vi "SelectOPCTags.GetChannelInfo.vi"(8 "error in (no error)":errorcluster, 10 "Item URL":string, 11 "OPC UA client refnum in":refnum<k21>) -> (0 "error out":errorcluster, 1 "Setings":T1={"Settings"={"name"="", "node type"=enum."Other", "DataType"=1, "access"=enum."Null", "description"=""}, "Array Size"=0} {"Settings"."DataType" items=["Boolean"=1, "SByte"=2, "Byte"=3, "Int16"=4, "UInt16"=5, "Int32"=6, "UInt32"=7, "Int64"=8, "UInt64"=9, "Float"=10, "Double"=11, "String"=12, "DateTime"=13, "ByteString"=15, "Array of Boolean"=101, "Array of SByte"=102, "Array of Byte"=103, "Array of Int16"=104, "Array of UInt16"=105, "Array of Int32"=106, "Array of UInt32"=107, "Array of Int64"=108, "Array of UInt64"=109, "Array of Float"=110, "Array of Double"=111, "Array of String"=112, "Array of DateTime"=113, "Array of ByteString"=115]}, 2 "Item URL out":string, 3 "OPC UA client refnum out":refnum<k21>, 4 "Use":bool)   [LabVIEW 2019, in "OPC UA Client System Explorer.lvlib"]
uses:
  OPC UA Client System Explorer.lvlib
  Types/Tag.TreeSettings.ctl
  <vilib>/OPCUA/NI OPC UA Client.lvlib
  <vilib>/OPCUA/client/internal/Read Double Array.vi
  <vilib>/OPCUA/client/internal/Read Float Array.vi
  <vilib>/OPCUA/client/internal/Read UInt32 Array.vi
  <vilib>/OPCUA/client/internal/Read Int32 Array.vi
  <vilib>/OPCUA/client/internal/Read UInt16 Array.vi
  <vilib>/OPCUA/client/internal/Read Int16 Array.vi
  <vilib>/OPCUA/client/internal/Read Byte Array.vi
  <vilib>/OPCUA/client/internal/Read SByte Array.vi
  <vilib>/OPCUA/client/internal/Read Bool Array.vi
  <vilib>/OPCUA/client/internal/Read UInt64 Array.vi
  <vilib>/OPCUA/client/internal/Read Int64 Array.vi
  <vilib>/OPCUA/client/internal/Read DateTime Array.vi
  <vilib>/OPCUA/client/internal/Read ByteString.vi
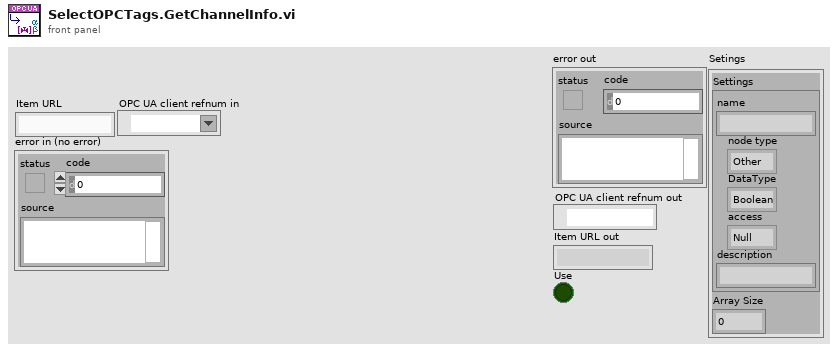
[diagram p1: front panel]
types:
  T1 = typedef "OPC UA Client System Explorer.lvlib/Tag.TreeSettings.ctl" = cluster{"Settings":cluster{"name":string, "node type":enum32{"Other", "Folder", "Item/Property"}, "DataType":u32, "access":enum16{"Null", "Read", "Write", "Read&Write"}, "description":string}, "Array Size":i32}
  T2 = typedef "Data Type Indicator.ctl" = u16
  T3 = cluster{"name":string, "node class":u16, "data type":T2, "access":enum16{"Null", "Read", "Write", "Read&Write"}, "description":string}
  T4 = typedef "OPC UA Client Refnum.ctl" = refnum<k21>
  T5 = typedef "OPC UA StatusCode.ctl" = u32
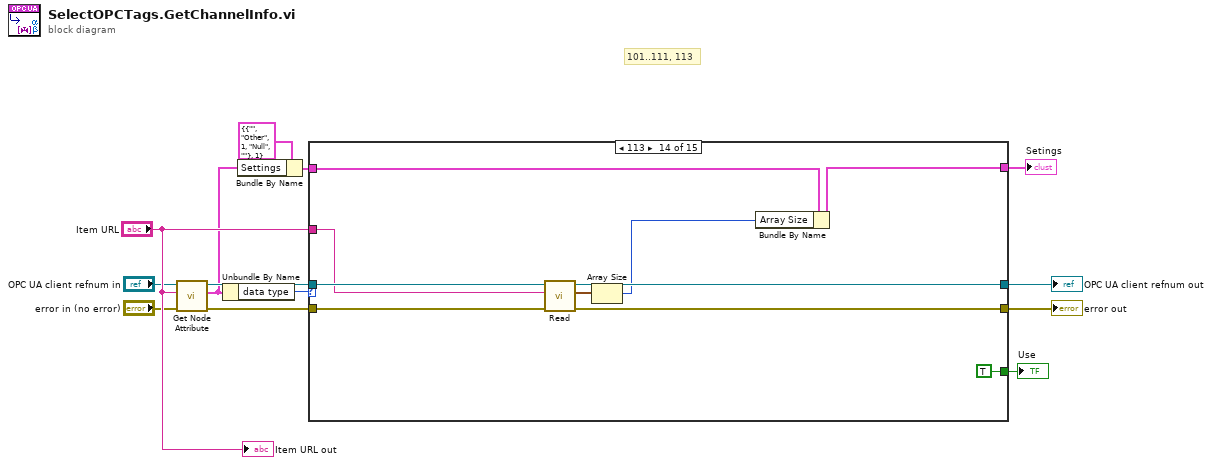
[diagram p0: block diagram]
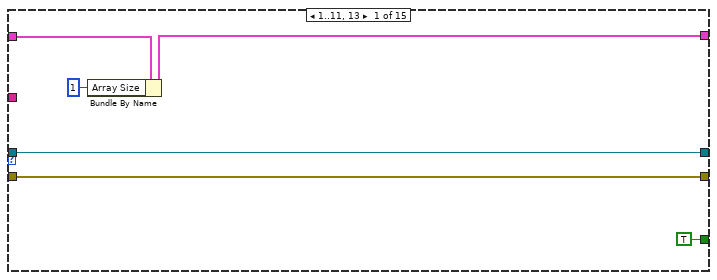
[diagram p2: hidden frame]
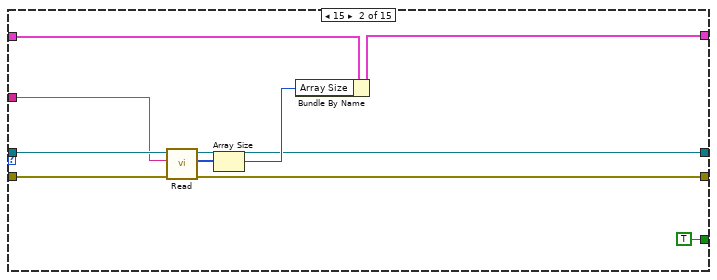
[diagram p3: hidden frame]
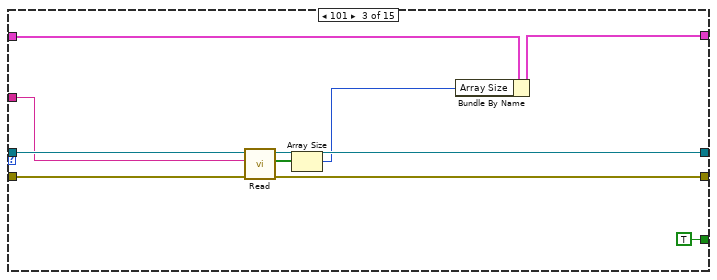
[diagram p4: hidden frame]
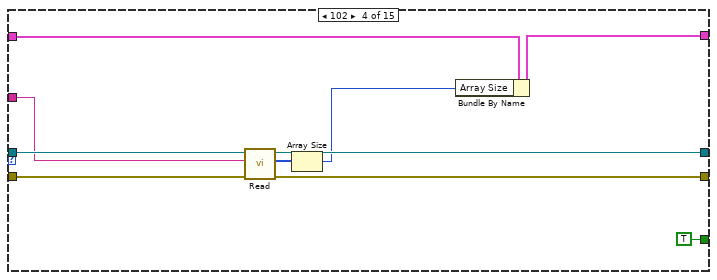
[diagram p5: hidden frame]
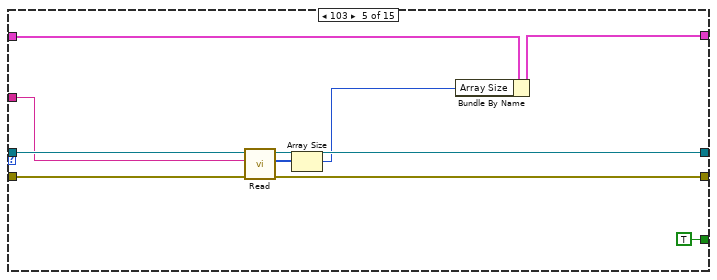
[diagram p6: hidden frame]
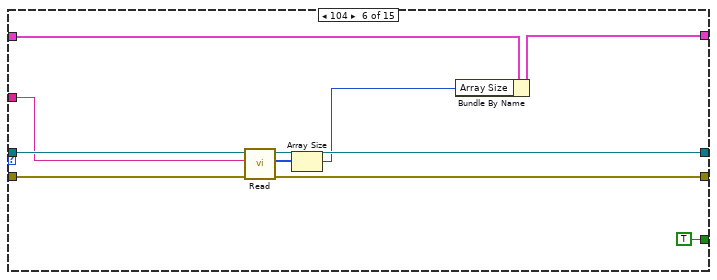
[diagram p7: hidden frame]
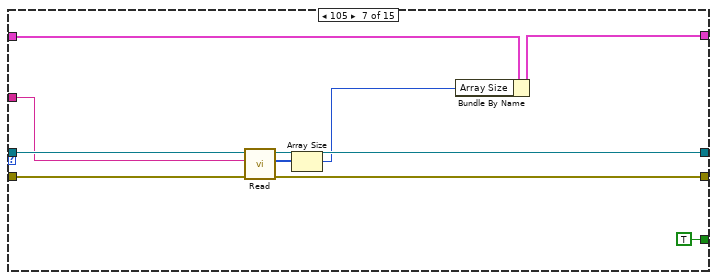
[diagram p8: hidden frame]
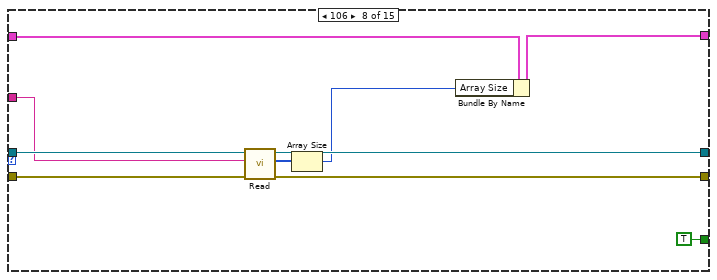
[diagram p9: hidden frame]
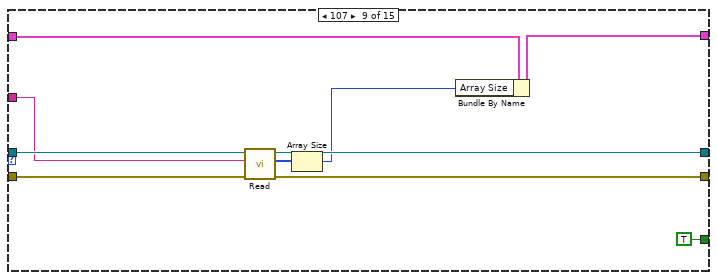
[diagram p10: hidden frame]
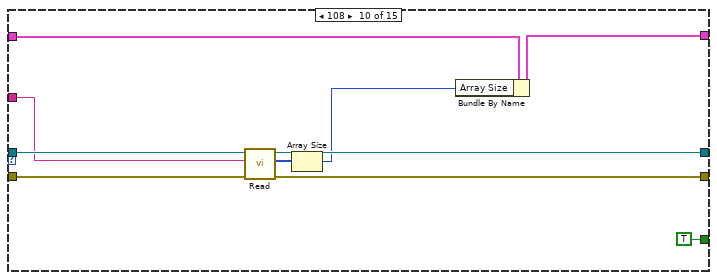
[diagram p11: hidden frame]
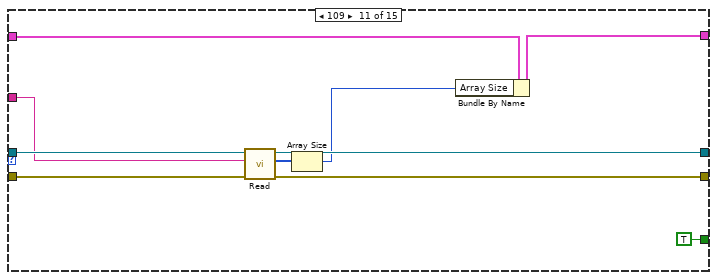
[diagram p12: hidden frame]
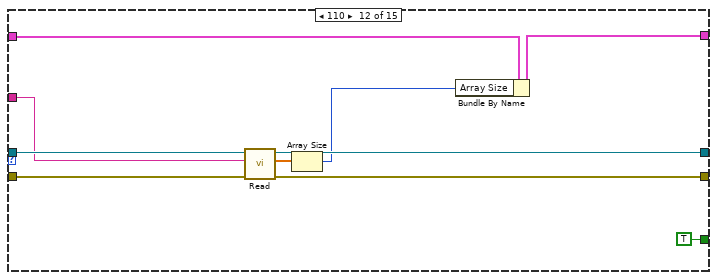
[diagram p13: hidden frame]
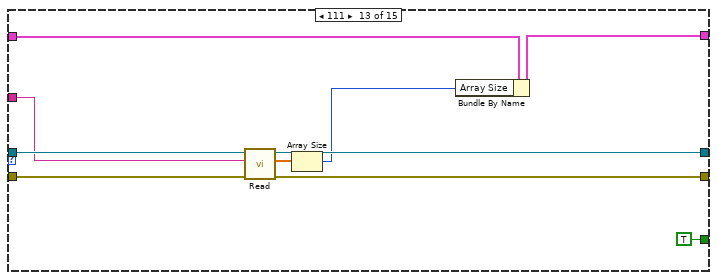
[diagram p14: hidden frame]
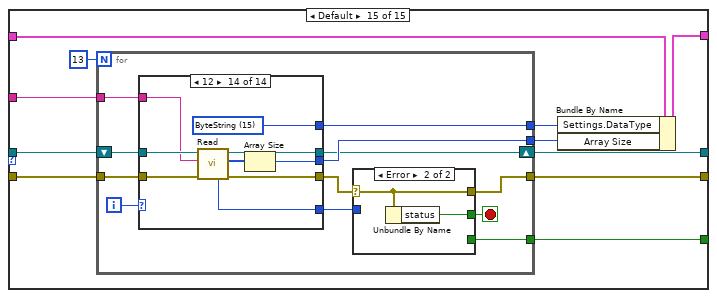
[diagram p15: hidden frame]
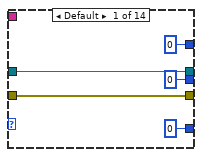
[diagram p16: hidden frame]
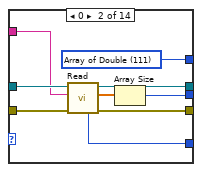
[diagram p17: hidden frame]
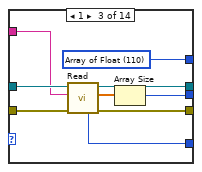
[diagram p18: hidden frame]
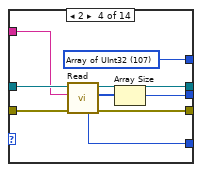
[diagram p19: hidden frame]
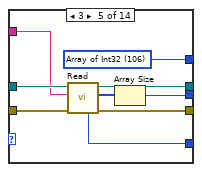
[diagram p20: hidden frame]
diagram:
  # "101..111, 113"
  n1 = call <vilib>:"Get Node Attribute.vi"("error in (no error)"="error in (no error)", "node ID"="Item URL", "OPC UA client refnum in"="OPC UA client refnum in") -> ("error out"=w6:errorcluster, "node attribute"=w4:T3, "OPC UA client refnum out"=w5:T4)  [unwired: 5 in, 1 out]
  n2 = Unbundle By Name(w4) -> ("data type"=w10:T2)
  n3 = Bundle By Name(cluster=T1 {"Settings"={"name"="", "node type"=enum."Other", "DataType"=1, "access"=enum."Null", "description"=""}, "Array Size"=1}, "Settings"=w4) -> (w9:T1)
  n4 = case shown="113" w10 {
    tunnel: [w16 w20 w34 w44 w54 w64 w74 w84 w94 w104 w114 w124 w134 w144 w152] -> w13
    tunnel: [w17 w21 w32 w42 w52 w62 w72 w82 w92 w102 w112 w122 w132 w142 w151] -> w12
    tunnel: w6 -> [w16 w25 w35 w45 w55 w65 w75 w85 w95 w105 w115 w125 w135 w145 w157]
    tunnel: w5 -> [w17 w24 w33 w43 w53 w63 w73 w83 w93 w103 w113 w123 w133 w143 w155]
    tunnel: "Item URL" -> [_ w23 w30 w40 w50 w60 w70 w80 w90 w100 w110 w120 w130 w140 w156]
    tunnel: w9 -> [w19 w29 w39 w49 w59 w69 w79 w89 w99 w109 w119 w129 w139 w149 w160]
    tunnel: [w18 w28 w38 w48 w58 w68 w78 w88 w98 w108 w118 w128 w138 w148 w159] -> w3
    tunnel: [TRUE ("status") TRUE ("status") TRUE ("status") TRUE ("status") TRUE ("status") TRUE ("status") TRUE ("status") TRUE ("status") TRUE ("status") TRUE ("status") TRUE ("status") TRUE ("status") TRUE ("status") TRUE ("status") w150] -> w2
    frame 1..11, 13 {
      n5 = Bundle By Name(cluster=w19, "Array Size"=1) -> (w18:T1)
    }
    frame 15 {
      n6 = call-poly <vilib>:"Read.vi"("error in (no error)"=w25, "node ID"=w23, "OPC UA client refnum in"=w24) -> ("error out"=w20:errorcluster, "value"=w26:u8[], "OPC UA client refnum out"=w21:T4)  [unwired: 4 in, 2 out]
      n7 = Array Size(array=w26) -> (size(s)=w22:i32)
      n8 = Bundle By Name(cluster=w29, "Array Size"=w22) -> (w28:T1)
    }
    frame 101 {
      n9 = call-poly <vilib>:"Read.vi"("error in (no error)"=w35, "node ID"=w30, "OPC UA client refnum in"=w33) -> ("error out"=w34:errorcluster, "values"=w36:bool[], "OPC UA client refnum out"=w32:T4)  [unwired: 4 in, 2 out]
      n10 = Array Size(array=w36) -> (size(s)=w31:i32)
      n11 = Bundle By Name(cluster=w39, "Array Size"=w31) -> (w38:T1)
    }
    frame 102 {
      n12 = call-poly <vilib>:"Read.vi"("error in (no error)"=w45, "node ID"=w40, "OPC UA client refnum in"=w43) -> ("error out"=w44:errorcluster, "values"=w46:i8[], "OPC UA client refnum out"=w42:T4)  [unwired: 4 in, 2 out]
      n13 = Array Size(array=w46) -> (size(s)=w41:i32)
      n14 = Bundle By Name(cluster=w49, "Array Size"=w41) -> (w48:T1)
    }
    frame 103 {
      n15 = call-poly <vilib>:"Read.vi"("error in (no error)"=w55, "node ID"=w50, "OPC UA client refnum in"=w53) -> ("error out"=w54:errorcluster, "values"=w56:u8[], "OPC UA client refnum out"=w52:T4)  [unwired: 4 in, 2 out]
      n16 = Array Size(array=w56) -> (size(s)=w51:i32)
      n17 = Bundle By Name(cluster=w59, "Array Size"=w51) -> (w58:T1)
    }
    frame 104 {
      n18 = call-poly <vilib>:"Read.vi"("error in (no error)"=w65, "node ID"=w60, "OPC UA client refnum in"=w63) -> ("error out"=w64:errorcluster, "values"=w66:i16[], "OPC UA client refnum out"=w62:T4)  [unwired: 4 in, 2 out]
      n19 = Array Size(array=w66) -> (size(s)=w61:i32)
      n20 = Bundle By Name(cluster=w69, "Array Size"=w61) -> (w68:T1)
    }
    frame 105 {
      n21 = call-poly <vilib>:"Read.vi"("error in (no error)"=w75, "node ID"=w70, "OPC UA client refnum in"=w73) -> ("error out"=w74:errorcluster, "values"=w76:u16[], "OPC UA client refnum out"=w72:T4)  [unwired: 4 in, 2 out]
      n22 = Array Size(array=w76) -> (size(s)=w71:i32)
      n23 = Bundle By Name(cluster=w79, "Array Size"=w71) -> (w78:T1)
    }
    frame 106 {
      n24 = call-poly <vilib>:"Read.vi"("error in (no error)"=w85, "node ID"=w80, "OPC UA client refnum in"=w83) -> ("error out"=w84:errorcluster, "values"=w86:i32[], "OPC UA client refnum out"=w82:T4)  [unwired: 4 in, 2 out]
      n25 = Array Size(array=w86) -> (size(s)=w81:i32)
      n26 = Bundle By Name(cluster=w89, "Array Size"=w81) -> (w88:T1)
    }
    frame 107 {
      n27 = call-poly <vilib>:"Read.vi"("error in (no error)"=w95, "node ID"=w90, "OPC UA client refnum in"=w93) -> ("error out"=w94:errorcluster, "values"=w96:u32[], "OPC UA client refnum out"=w92:T4)  [unwired: 4 in, 2 out]
      n28 = Array Size(array=w96) -> (size(s)=w91:i32)
      n29 = Bundle By Name(cluster=w99, "Array Size"=w91) -> (w98:T1)
    }
    frame 108 {
      n30 = call-poly <vilib>:"Read.vi"("error in (no error)"=w105, "node ID"=w100, "OPC UA client refnum in"=w103) -> ("error out"=w104:errorcluster, "values"=w106:i64[], "OPC UA client refnum out"=w102:T4)  [unwired: 4 in, 2 out]
      n31 = Array Size(array=w106) -> (size(s)=w101:i32)
      n32 = Bundle By Name(cluster=w109, "Array Size"=w101) -> (w108:T1)
    }
    frame 109 {
      n33 = call-poly <vilib>:"Read.vi"("error in (no error)"=w115, "node ID"=w110, "OPC UA client refnum in"=w113) -> ("error out"=w114:errorcluster, "values"=w116:u64[], "OPC UA client refnum out"=w112:T4)  [unwired: 4 in, 2 out]
      n34 = Array Size(array=w116) -> (size(s)=w111:i32)
      n35 = Bundle By Name(cluster=w119, "Array Size"=w111) -> (w118:T1)
    }
    frame 110 {
      n36 = call-poly <vilib>:"Read.vi"("error in (no error)"=w125, "node ID"=w120, "OPC UA client refnum in"=w123) -> ("error out"=w124:errorcluster, "values"=w126:sgl[], "OPC UA client refnum out"=w122:T4)  [unwired: 4 in, 2 out]
      n37 = Array Size(array=w126) -> (size(s)=w121:i32)
      n38 = Bundle By Name(cluster=w129, "Array Size"=w121) -> (w128:T1)
    }
    frame 111 {
      n39 = call-poly <vilib>:"Read.vi"("error in (no error)"=w135, "node ID"=w130, "OPC UA client refnum in"=w133) -> ("error out"=w134:errorcluster, "values"=w136:dbl[], "OPC UA client refnum out"=w132:T4)  [unwired: 4 in, 2 out]
      n40 = Array Size(array=w136) -> (size(s)=w131:i32)
      n41 = Bundle By Name(cluster=w139, "Array Size"=w131) -> (w138:T1)
    }
    frame 113 {
      n42 = call-poly <vilib>:"Read.vi"("error in (no error)"=w145, "node ID"=w140, "OPC UA client refnum in"=w143) -> ("error out"=w144:errorcluster, "values"=w146:timestamp[], "OPC UA client refnum out"=w142:T4)  [unwired: 4 in, 2 out]
      n43 = Array Size(array=w146) -> (size(s)=w141:i32)
      n44 = Bundle By Name(cluster=w149, "Array Size"=w141) -> (w148:T1)
    }
    frame Default {
      n45 = for {
        N: 13 -> [_]
        tunnel: w157 -> [w172]
        tunnel: w156 -> [w170]
        tunnel: [w167] -> w152
        tunnel: [w165] -> w153
        tunnel: [w164] -> w154
        shift-right: [w163] -> w151
        shift-left: w155 -> [w171]
        tunnel: [w161] -> w150
        i -> [w166]
        stop <- w162 stop-if-true
        n46 = case shown="12" w166 {
          tunnel: w172 -> [w175 w186 w195 w204 w213 w222 w231 w240 w249 w258 w267 w276 w285 w294]
          tunnel: w171 -> [w173 w185 w194 w203 w212 w221 w230 w239 w248 w257 w266 w275 w284 w293]
          tunnel: w170 -> [_ w184 w193 w202 w211 w220 w229 w238 w247 w256 w265 w274 w283 w292]
          tunnel: [w175 w183 w192 w201 w210 w219 w228 w237 w246 w255 w264 w273 w282 w291] -> w169
          tunnel: [u32 0 ("status") w182 w191 w200 w209 w218 w227 w236 w245 w254 w263 w272 w281 w290] -> w168
          tunnel: [u32 0 ("DataType") w180 w189 w198 w207 w216 w225 w234 w243 w252 w261 w270 w279 w288] -> w164
          tunnel: [0 w179 w188 w197 w206 w215 w224 w233 w242 w251 w260 w269 w278 w287] -> w165
          tunnel: [w173 w178 w187 w196 w205 w214 w223 w232 w241 w250 w259 w268 w277 w286] -> w163
          frame Default {
          }
          frame 0 {
            w180 = u32 111 items=["Boolean"=1, "SByte"=2, "Byte"=3, "Int16"=4, "UInt16"=5, "Int32"=6, "UInt32"=7, "Int64"=8, "UInt64"=9, "Float"=10, "Double"=11, "String"=12, "DateTime"=13, "ByteString"=15, "Array of Boolean"=101, "Array of SByte"=102, "Array of Byte"=103, "Array of Int16"=104, "Array of UInt16"=105, "Array of Int32"=106, "Array of UInt32"=107, "Array of Int64"=108, "Array of UInt64"=109, "Array of Float"=110, "Array of Double"=111, "Array of String"=112, "Array of DateTime"=113, "Array of ByteString"=115] ("DataType")
            n47 = call-poly <vilib>:"Read.vi"("error in (no error)"=w186, "node ID"=w184, "OPC UA client refnum in"=w185) -> ("error out"=w183:errorcluster, "values"=w181:dbl[], "OPC UA client refnum out"=w178:T4, "status"=w182:T5)  [unwired: 4 in, 1 out]
            n48 = Array Size(array=w181) -> (size(s)=w179:i32)
          }
          frame 1 {
            w189 = u32 110 items=["Boolean"=1, "SByte"=2, "Byte"=3, "Int16"=4, "UInt16"=5, "Int32"=6, "UInt32"=7, "Int64"=8, "UInt64"=9, "Float"=10, "Double"=11, "String"=12, "DateTime"=13, "ByteString"=15, "Array of Boolean"=101, "Array of SByte"=102, "Array of Byte"=103, "Array of Int16"=104, "Array of UInt16"=105, "Array of Int32"=106, "Array of UInt32"=107, "Array of Int64"=108, "Array of UInt64"=109, "Array of Float"=110, "Array of Double"=111, "Array of String"=112, "Array of DateTime"=113, "Array of ByteString"=115] ("DataType")
            n49 = call-poly <vilib>:"Read.vi"("error in (no error)"=w195, "node ID"=w193, "OPC UA client refnum in"=w194) -> ("error out"=w192:errorcluster, "values"=w190:sgl[], "OPC UA client refnum out"=w187:T4, "status"=w191:T5)  [unwired: 4 in, 1 out]
            n50 = Array Size(array=w190) -> (size(s)=w188:i32)
          }
          frame 2 {
            w198 = u32 107 items=["Boolean"=1, "SByte"=2, "Byte"=3, "Int16"=4, "UInt16"=5, "Int32"=6, "UInt32"=7, "Int64"=8, "UInt64"=9, "Float"=10, "Double"=11, "String"=12, "DateTime"=13, "ByteString"=15, "Array of Boolean"=101, "Array of SByte"=102, "Array of Byte"=103, "Array of Int16"=104, "Array of UInt16"=105, "Array of Int32"=106, "Array of UInt32"=107, "Array of Int64"=108, "Array of UInt64"=109, "Array of Float"=110, "Array of Double"=111, "Array of String"=112, "Array of DateTime"=113, "Array of ByteString"=115] ("DataType")
            n51 = call-poly <vilib>:"Read.vi"("error in (no error)"=w204, "node ID"=w202, "OPC UA client refnum in"=w203) -> ("error out"=w201:errorcluster, "values"=w199:u32[], "OPC UA client refnum out"=w196:T4, "status"=w200:T5)  [unwired: 4 in, 1 out]
            n52 = Array Size(array=w199) -> (size(s)=w197:i32)
          }
          frame 3 {
            w207 = u32 106 items=["Boolean"=1, "SByte"=2, "Byte"=3, "Int16"=4, "UInt16"=5, "Int32"=6, "UInt32"=7, "Int64"=8, "UInt64"=9, "Float"=10, "Double"=11, "String"=12, "DateTime"=13, "ByteString"=15, "Array of Boolean"=101, "Array of SByte"=102, "Array of Byte"=103, "Array of Int16"=104, "Array of UInt16"=105, "Array of Int32"=106, "Array of UInt32"=107, "Array of Int64"=108, "Array of UInt64"=109, "Array of Float"=110, "Array of Double"=111, "Array of String"=112, "Array of DateTime"=113, "Array of ByteString"=115] ("DataType")
            n53 = call-poly <vilib>:"Read.vi"("error in (no error)"=w213, "node ID"=w211, "OPC UA client refnum in"=w212) -> ("error out"=w210:errorcluster, "values"=w208:i32[], "OPC UA client refnum out"=w205:T4, "status"=w209:T5)  [unwired: 4 in, 1 out]
            n54 = Array Size(array=w208) -> (size(s)=w206:i32)
          }
          frame 4 {
            w216 = u32 105 items=["Boolean"=1, "SByte"=2, "Byte"=3, "Int16"=4, "UInt16"=5, "Int32"=6, "UInt32"=7, "Int64"=8, "UInt64"=9, "Float"=10, "Double"=11, "String"=12, "DateTime"=13, "ByteString"=15, "Array of Boolean"=101, "Array of SByte"=102, "Array of Byte"=103, "Array of Int16"=104, "Array of UInt16"=105, "Array of Int32"=106, "Array of UInt32"=107, "Array of Int64"=108, "Array of UInt64"=109, "Array of Float"=110, "Array of Double"=111, "Array of String"=112, "Array of DateTime"=113, "Array of ByteString"=115] ("DataType")
            n55 = call-poly <vilib>:"Read.vi"("error in (no error)"=w222, "node ID"=w220, "OPC UA client refnum in"=w221) -> ("error out"=w219:errorcluster, "values"=w217:u16[], "OPC UA client refnum out"=w214:T4, "status"=w218:T5)  [unwired: 4 in, 1 out]
            n56 = Array Size(array=w217) -> (size(s)=w215:i32)
          }
          frame 5 {
            w225 = u32 104 items=["Boolean"=1, "SByte"=2, "Byte"=3, "Int16"=4, "UInt16"=5, "Int32"=6, "UInt32"=7, "Int64"=8, "UInt64"=9, "Float"=10, "Double"=11, "String"=12, "DateTime"=13, "ByteString"=15, "Array of Boolean"=101, "Array of SByte"=102, "Array of Byte"=103, "Array of Int16"=104, "Array of UInt16"=105, "Array of Int32"=106, "Array of UInt32"=107, "Array of Int64"=108, "Array of UInt64"=109, "Array of Float"=110, "Array of Double"=111, "Array of String"=112, "Array of DateTime"=113, "Array of ByteString"=115] ("DataType")
            n57 = call-poly <vilib>:"Read.vi"("error in (no error)"=w231, "node ID"=w229, "OPC UA client refnum in"=w230) -> ("error out"=w228:errorcluster, "values"=w226:i16[], "OPC UA client refnum out"=w223:T4, "status"=w227:T5)  [unwired: 4 in, 1 out]
            n58 = Array Size(array=w226) -> (size(s)=w224:i32)
          }
          frame 6 {
            w234 = u32 103 items=["Boolean"=1, "SByte"=2, "Byte"=3, "Int16"=4, "UInt16"=5, "Int32"=6, "UInt32"=7, "Int64"=8, "UInt64"=9, "Float"=10, "Double"=11, "String"=12, "DateTime"=13, "ByteString"=15, "Array of Boolean"=101, "Array of SByte"=102, "Array of Byte"=103, "Array of Int16"=104, "Array of UInt16"=105, "Array of Int32"=106, "Array of UInt32"=107, "Array of Int64"=108, "Array of UInt64"=109, "Array of Float"=110, "Array of Double"=111, "Array of String"=112, "Array of DateTime"=113, "Array of ByteString"=115] ("DataType")
            n59 = call-poly <vilib>:"Read.vi"("error in (no error)"=w240, "node ID"=w238, "OPC UA client refnum in"=w239) -> ("error out"=w237:errorcluster, "values"=w235:u8[], "OPC UA client refnum out"=w232:T4, "status"=w236:T5)  [unwired: 4 in, 1 out]
            n60 = Array Size(array=w235) -> (size(s)=w233:i32)
          }
          frame 7 {
            w243 = u32 102 items=["Boolean"=1, "SByte"=2, "Byte"=3, "Int16"=4, "UInt16"=5, "Int32"=6, "UInt32"=7, "Int64"=8, "UInt64"=9, "Float"=10, "Double"=11, "String"=12, "DateTime"=13, "ByteString"=15, "Array of Boolean"=101, "Array of SByte"=102, "Array of Byte"=103, "Array of Int16"=104, "Array of UInt16"=105, "Array of Int32"=106, "Array of UInt32"=107, "Array of Int64"=108, "Array of UInt64"=109, "Array of Float"=110, "Array of Double"=111, "Array of String"=112, "Array of DateTime"=113, "Array of ByteString"=115] ("DataType")
            n61 = call-poly <vilib>:"Read.vi"("error in (no error)"=w249, "node ID"=w247, "OPC UA client refnum in"=w248) -> ("error out"=w246:errorcluster, "values"=w244:i8[], "OPC UA client refnum out"=w241:T4, "status"=w245:T5)  [unwired: 4 in, 1 out]
            n62 = Array Size(array=w244) -> (size(s)=w242:i32)
          }
          frame 8 {
            w252 = u32 101 items=["Boolean"=1, "SByte"=2, "Byte"=3, "Int16"=4, "UInt16"=5, "Int32"=6, "UInt32"=7, "Int64"=8, "UInt64"=9, "Float"=10, "Double"=11, "String"=12, "DateTime"=13, "ByteString"=15, "Array of Boolean"=101, "Array of SByte"=102, "Array of Byte"=103, "Array of Int16"=104, "Array of UInt16"=105, "Array of Int32"=106, "Array of UInt32"=107, "Array of Int64"=108, "Array of UInt64"=109, "Array of Float"=110, "Array of Double"=111, "Array of String"=112, "Array of DateTime"=113, "Array of ByteString"=115] ("DataType")
            n63 = call-poly <vilib>:"Read.vi"("error in (no error)"=w258, "node ID"=w256, "OPC UA client refnum in"=w257) -> ("error out"=w255:errorcluster, "values"=w253:bool[], "OPC UA client refnum out"=w250:T4, "status"=w254:T5)  [unwired: 4 in, 1 out]
            n64 = Array Size(array=w253) -> (size(s)=w251:i32)
          }
          frame 9 {
            w261 = u32 109 items=["Boolean"=1, "SByte"=2, "Byte"=3, "Int16"=4, "UInt16"=5, "Int32"=6, "UInt32"=7, "Int64"=8, "UInt64"=9, "Float"=10, "Double"=11, "String"=12, "DateTime"=13, "ByteString"=15, "Array of Boolean"=101, "Array of SByte"=102, "Array of Byte"=103, "Array of Int16"=104, "Array of UInt16"=105, "Array of Int32"=106, "Array of UInt32"=107, "Array of Int64"=108, "Array of UInt64"=109, "Array of Float"=110, "Array of Double"=111, "Array of String"=112, "Array of DateTime"=113, "Array of ByteString"=115] ("DataType")
            n65 = call-poly <vilib>:"Read.vi"("error in (no error)"=w267, "node ID"=w265, "OPC UA client refnum in"=w266) -> ("error out"=w264:errorcluster, "values"=w262:u64[], "OPC UA client refnum out"=w259:T4, "status"=w263:T5)  [unwired: 4 in, 1 out]
            n66 = Array Size(array=w262) -> (size(s)=w260:i32)
          }
          frame 10 {
            w270 = u32 108 items=["Boolean"=1, "SByte"=2, "Byte"=3, "Int16"=4, "UInt16"=5, "Int32"=6, "UInt32"=7, "Int64"=8, "UInt64"=9, "Float"=10, "Double"=11, "String"=12, "DateTime"=13, "ByteString"=15, "Array of Boolean"=101, "Array of SByte"=102, "Array of Byte"=103, "Array of Int16"=104, "Array of UInt16"=105, "Array of Int32"=106, "Array of UInt32"=107, "Array of Int64"=108, "Array of UInt64"=109, "Array of Float"=110, "Array of Double"=111, "Array of String"=112, "Array of DateTime"=113, "Array of ByteString"=115] ("DataType")
            n67 = call-poly <vilib>:"Read.vi"("error in (no error)"=w276, "node ID"=w274, "OPC UA client refnum in"=w275) -> ("error out"=w273:errorcluster, "values"=w271:i64[], "OPC UA client refnum out"=w268:T4, "status"=w272:T5)  [unwired: 4 in, 1 out]
            n68 = Array Size(array=w271) -> (size(s)=w269:i32)
          }
          frame 11 {
            w279 = u32 113 items=["Boolean"=1, "SByte"=2, "Byte"=3, "Int16"=4, "UInt16"=5, "Int32"=6, "UInt32"=7, "Int64"=8, "UInt64"=9, "Float"=10, "Double"=11, "String"=12, "DateTime"=13, "ByteString"=15, "Array of Boolean"=101, "Array of SByte"=102, "Array of Byte"=103, "Array of Int16"=104, "Array of UInt16"=105, "Array of Int32"=106, "Array of UInt32"=107, "Array of Int64"=108, "Array of UInt64"=109, "Array of Float"=110, "Array of Double"=111, "Array of String"=112, "Array of DateTime"=113, "Array of ByteString"=115] ("DataType")
            n69 = call-poly <vilib>:"Read.vi"("error in (no error)"=w285, "node ID"=w283, "OPC UA client refnum in"=w284) -> ("error out"=w282:errorcluster, "values"=w280:timestamp[], "OPC UA client refnum out"=w277:T4, "status"=w281:T5)  [unwired: 4 in, 1 out]
            n70 = Array Size(array=w280) -> (size(s)=w278:i32)
          }
          frame 12 {
            w288 = u32 15 items=["Boolean"=1, "SByte"=2, "Byte"=3, "Int16"=4, "UInt16"=5, "Int32"=6, "UInt32"=7, "Int64"=8, "UInt64"=9, "Float"=10, "Double"=11, "String"=12, "DateTime"=13, "ByteString"=15, "Array of Boolean"=101, "Array of SByte"=102, "Array of Byte"=103, "Array of Int16"=104, "Array of UInt16"=105, "Array of Int32"=106, "Array of UInt32"=107, "Array of Int64"=108, "Array of UInt64"=109, "Array of Float"=110, "Array of Double"=111, "Array of String"=112, "Array of DateTime"=113, "Array of ByteString"=115] ("DataType")
            n71 = call-poly <vilib>:"Read.vi"("error in (no error)"=w294, "node ID"=w292, "OPC UA client refnum in"=w293) -> ("error out"=w291:errorcluster, "value"=w289:u8[], "OPC UA client refnum out"=w286:T4, "status"=w290:T5)  [unwired: 4 in, 1 out]
            n72 = Array Size(array=w289) -> (size(s)=w287:i32)
          }
        }
        n73 = case shown="Error" w169 {
          selector: w169 -> [w296 w299]
          tunnel: w168 -> [w298 _]
          tunnel: [w295 w300] -> w162
          tunnel: [w296 w299] -> w167
          tunnel: [w295 _] -> w161
          frame No Error {
            w297 = u32 0 items=["Good"=0, "Bad_AttributeIdInvalid"=2153906176, "Bad_BrowseDirectionInvalid"=2152529920, "Bad_BrowseNameInvalid"=2153775104, "Bad_ContentFilterInvalid"=2152202240, "Bad_ContinuationPointInvalid"=2152333312, "Bad_DataEncodingInvalid"=2151153664, "Bad_DataEncodingUnsupported"=2151219200, "Bad_EventFilterInvalid"=2152136704, "Bad_FilterNotAllowed"=2152005632, "Bad_FilterOperandInvalid"=2160132096, "Bad_HistoryOperationInvalid"=2154889216, "Bad_HistoryOperationUnsupported"=2154954752, "Bad_IndexRangeInvalid"=2151022592, "Bad_IndexRangeNoData"=2151088128, "Bad_MonitoredItemFilterInvalid"=2151874560, "Bad_MonitoredItemFilterUnsupported"=2151940096, "Bad_MonitoredItemIdInvalid"=2151809024, "Bad_MonitoringModeInvalid"=2151743488, "Bad_NoCommunication"=2150694912, "Bad_NoContinuationPoints"=2152398848, "Bad_NodeClassInvalid"=2153709568, "Bad_NodeIdInvalid"=2150825984, "Bad_NodeIdUnknown"=2150891520, "Bad_NoDeleteRights"=2154364928, "Bad_NodeNotInView"=2152595456, "Bad_NotFound"=2151546880, "Bad_NotImplemented"=2151677952, "Bad_NotReadable"=2151284736, "Bad_NotSupported"=2151481344, "Bad_NotWritable"=2151350272, "Bad_ObjectDeleted"=2151612416, "Bad_OutOfRange"=2151415808, "Bad_ReferenceTypeIdInvalid"=2152464384, "Bad_SourceNodeIdInvalid"=2154037248, "Bad_StructureMissing"=2152071168, "Bad_TargetNodeIdInvalid"=2154102784, "Bad_TypeDefinitionInvalid"=2153971712, "Bad_TypeMismatch"=2155085824, "Bad_WaitingForInitialData"=2150760448] ("status")
            n74 = Equal?(x=w298, y=w297) -> (x = y?=w295:bool)
          }
          frame Error {
            n75 = Unbundle By Name(w299) -> ("status"=w300:bool)
          }
        }
      }
      n76 = Bundle By Name(cluster=w160, "Settings.DataType"=w154, "Array Size"=w153) -> (w159:T1)
    }
  }
  "error out" <- w13
  "OPC UA client refnum out" <- w12
  "Setings" <- w3
  "Use" <- w2
  "Item URL out" <- "Item URL"
